vi "read engine configuration.vi"(8 "error in":errorcluster, 11 "Engine Parent Editor Node in":refnum<class "Engine Parent Editor Node.lvclass">) -> (0 "error out":errorcluster, 2 "engine configuration":refnum<class "engine configuration.lvclass">, 3 "Engine Parent Editor Node out":refnum<class "Engine Parent Editor Node.lvclass">)   [LabVIEW 2013, in "PL Framework Configuration Tool.lvlib" / "Engine Parent Editor Node.lvclass"]
uses:
  Engine Parent Editor Node.lvclass
  <vilib>/NI/Module Execution Interface/Engine Configuration/engine configuration.lvclass
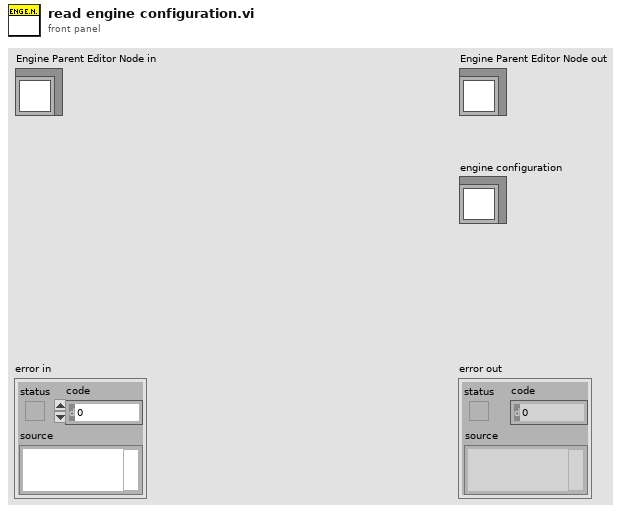
[diagram p1: front panel]
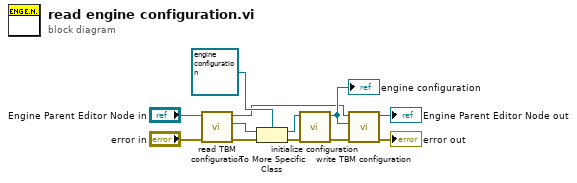
[diagram p0: block diagram]
diagram:
  n1 = call-dynamic "read TBM configuration.vi"("error in"="error in", "TBM Configuration Node in"="Engine Parent Editor Node in") -> ("error out"=w2:errorcluster, "configuration"=w3:refnum<class "TBM configuration.lvclass">, "TBM Configuration Node out"=w1:refnum<class "Engine Parent Editor Node.lvclass">)  [unwired: 7 in]
  n2 = To More Specific Class(target class=refnum<class "engine configuration.lvclass"> refnum ("engine configuration"), reference=w3, error in=w2) -> (specific class reference=w11:refnum<class "engine configuration.lvclass">, error out=w7:errorcluster)
  n3 = call-dynamic "initialize configuration.vi"("error in"=w7, "configuration in"=w11) -> ("error out"=w6:errorcluster, "configuration out"=w8:refnum<class "engine configuration.lvclass">)  [unwired: 7 in, 1 out]
  "engine configuration" <- w8
  n4 = call-dynamic "write TBM configuration.vi"("error in"=w6, "configuration"=w8, "TBM Configuration Node in"=w1) -> ("error out"=→"error out":errorcluster, "TBM Configuration Node out"=→"Engine Parent Editor Node out":refnum<class "Engine Parent Editor Node.lvclass">)  [unwired: 7 in]
